vi "tsapp_transmit_can_async.vi"(8 "Incorrect input (no errors)":errorcluster, 10 "TCAN":T1 {"AIsData" items=["Data Frame", "Remote Frame"]; "AIsStd" items=["Standard Frame", "Extended Frame"]; "AId" format="%x"; "AIdxchn" items=["CHN1", "CHN2", "CHN3", "CHN4", "CHN5", "CHN6", "CHN7", "CHN8", "CHN9", "CHN10", "CHN11", "CHN12", "CHN13", "CHN14", "CHN15", "CHN16", "CHN17", "CHN18", "CHN19", "CHN20", "CHN21", "CHN22", "CHN23", "CHN24", "CHN25", "CHN26", "CHN27", "CHN28", "CHN29", "CHN30", "CHN31", "CHN32"]}, 11 "Path input":path) -> (0 "error output":errorcluster, 2 "return":i32, 3 "Path output":path)   [LabVIEW 2014]
doc: "Function Introduction :\nSending CAN messages asynchronously\nCall location :\nSending CAN messages\ninput parameter :\nACAN: CAN packet. TLIBCAN data composition, please refer to chapter: TLIBCAN: Classical CAN\nData type. \nReturn value :\n==0: Sent successfully\nOther values: Sending failed, please refer to the error code for the reason of the failure"
uses:
  Typedef/TLibCAN.ctl
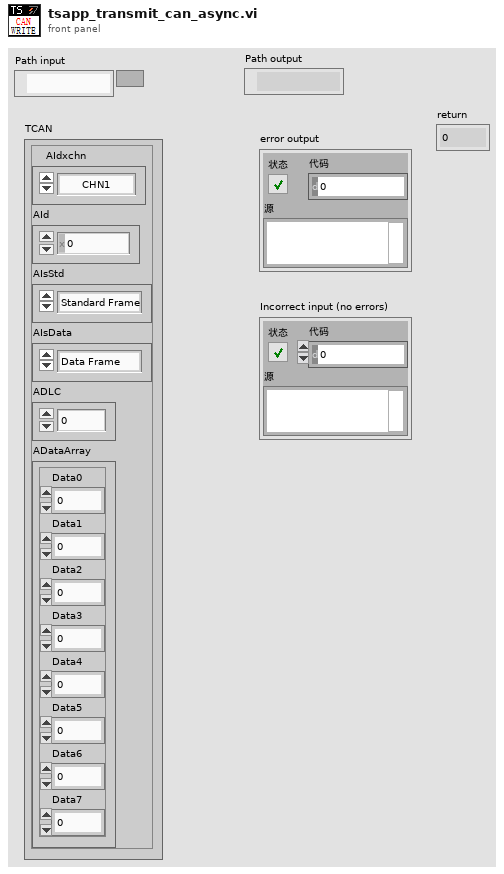
[diagram p1: front panel]
types:
  T1 = typedef "TLibCAN.ctl" = cluster{"AIdxchn":u8, "AId":i32, "AIsStd":u8, "AIsData":u8, "ADLC":u8, "ADataArray":cluster{"Data0":u8, "Data1":u8, "Data2":u8, "Data3":u8, "Data4":u8, "Data5":u8, "Data6":u8, "Data7":u8}}
  T2 = cluster{"FIdxChn":u8, "FProperties":u8, "FDLC":u8, "FReserved":u8, "FIdentifier":i32, "FTimeUS":u64, "FData":cluster{"Data0":u8, "Data1":u8, "Data2":u8, "Data3":u8, "Data4":u8, "Data5":u8, "Data6":u8, "Data7":u8}}
  T3 = cluster{"Data0":u8, "Data1":u8, "Data2":u8, "Data3":u8, "Data4":u8, "Data5":u8, "Data6":u8, "Data7":u8}
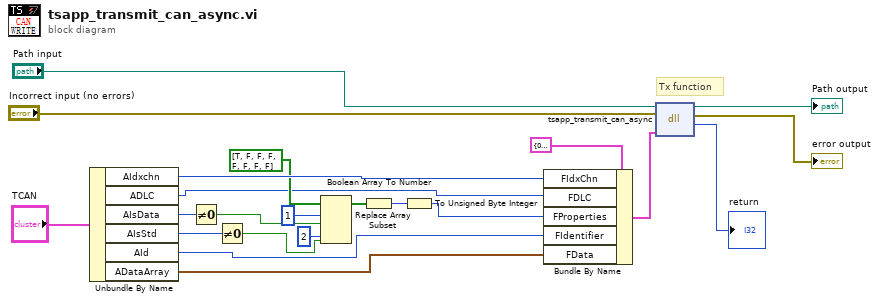
[diagram p0: block diagram]
diagram:
  # "Tx function"
  n1 = Unbundle By Name("TCAN") -> ("AIdxchn"=w13:u8, "ADLC"=w3:u8, "AIsData"=w12:u8, "AIsStd"=w11:u8, "AId"=w14:i32, "ADataArray"=w15:T3)
  n2 = Not Equal To 0?(x=w12) -> (x != 0?=w8:bool)
  n3 = Not Equal To 0?(x=w11) -> (x != 0?=w6:bool)
  n4 = Replace Array Subset(array=bool[] [TRUE, FALSE, FALSE, FALSE, FALSE, FALSE, FALSE, FALSE], new element #1=w8, index #1=1 ("索引"), new element #2=w6, index #2=2 ("索引")) -> (w5:bool[])
  n5 = Boolean Array To Number(Boolean array=w5) -> (number=w4:u32)
  n6 = To Unsigned Byte Integer(number=w4) -> (unsigned 8bit integer=w2:u8)
  n7 = Bundle By Name(cluster=T2 {"FIdxChn"=0, "FProperties"=0, "FDLC"=0, "FReserved"=0, "FIdentifier"=0, "FTimeUS"=0, "FData"={"Data0"=0, "Data1"=0, "Data2"=0, "Data3"=0, "Data4"=0, "Data5"=0, "Data6"=0, "Data7"=0}} ("簇"), "FIdxChn"=w13, "FDLC"=w3, "FProperties"=w2, "FIdentifier"=w14, "FData"=w15) -> (w17:T2)
  n8 = dll-call lib="C:/Users/Administrator/Desktop/TS_Can/Path/TSMaster.dll" fn="tsapp_transmit_can_async"(path in="Path input", error in="Incorrect input (no errors)", "ACAN"=w17) -> (path out=→"Path output":path, error out=→"error output":errorcluster, "tsapp_transmit_can_async"=→"return":i32)  [unwired: 2 in]
